vi "Period Trigged Timer（SRU）.vi"(5 "time (ms)":u32, 9 "reset":bool) -> (6 "Triggered":bool, 8 "time since last call":u32, 10 "timer value":u32)   [LabVIEW 2012, in "毫秒定时器.lvlib"]
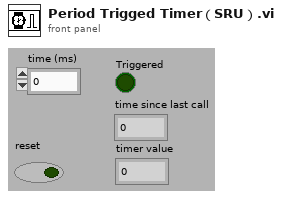
[diagram p1: front panel]
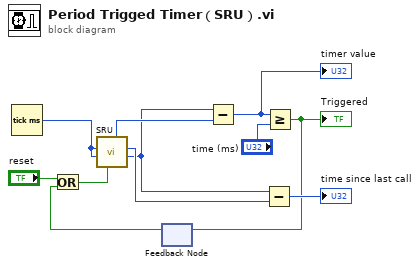
[diagram p0: block diagram]
diagram:
  n1 = Tick Count (ms)() -> (millisecond timer value=w6:u32)
  n2 = feedback #1() -> (w4:bool)  [unwired: 1 in]
  n3 = Or(x="reset", y=w4) -> (x .or. y?=w1:bool)
  n4 = call-poly "SRU.vi"("复位"=w1, "初始值"=w6, "输入"=w6) -> ("本次值"=w3:u32, "上次值"=w10:u32, "初始值"=w11:u32)  [unwired: 6 in]
  n5 = Subtract(x=w3, y=w11) -> (x-y=w2:u32)
  "timer value" <- w2
  n6 = Subtract(x=w3, y=w10) -> (x-y=→"time since last call":u32)
  n7 = Greater Or Equal?(x=w2, y="time (ms)") -> (x >= y?=w7:bool)
  "Triggered" <- w7
  n8 = feedback-in #1(w7) -> ()
